vi "Initialise Sound From File.vi"(8 "error in (no error)":errorcluster, 10 "Name":string, 11 "File":path) -> (0 "error out":errorcluster, 3 "Name In Cache":string)   [LabVIEW 2015, in "Resource Manager.lvclass"]
uses:
  Resource Manager.lvclass
  Resource Manager.lvclass/Resource Manager.ctl
  Globals.vi
  LabSDL2/Source/Libraries/LibSDL2_Mixer Wrapper/LibSDL2_Mixer.lvlib
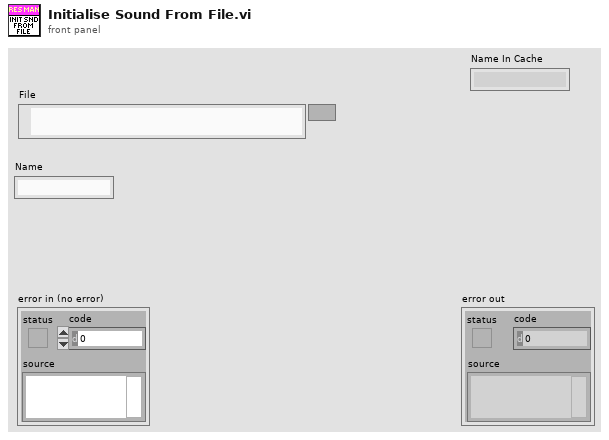
[diagram p1: front panel]
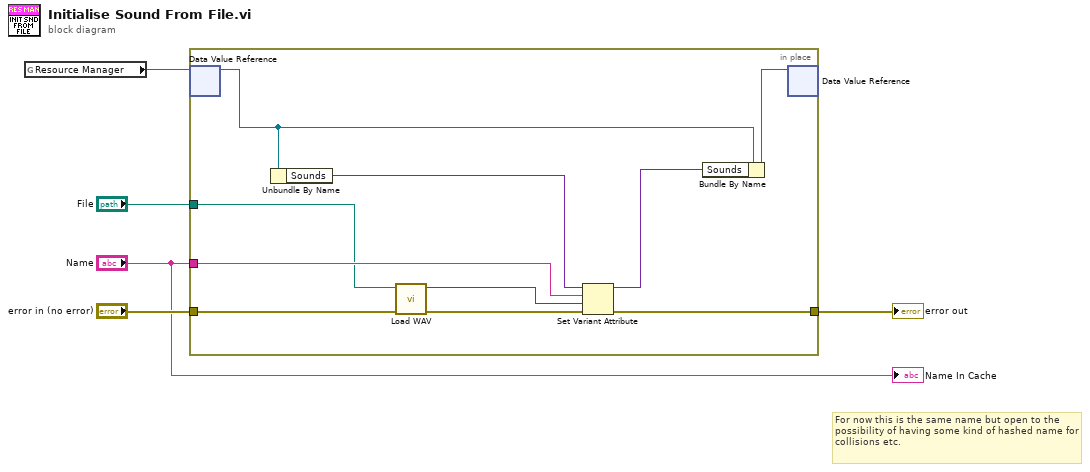
[diagram p0: block diagram]
diagram:
  # "For now this is the same name but open to the possibility of having some kind of hashed name for collisions etc."
  n1 = global read "Globals.vi" "Resource Manager"() -> (w1:refnum<data-value>)
  n2 = in-place {
    in-place-border: "File" -> [w7]
    in-place-border: "error in (no error)" -> [w9]
    in-place-border: [w14] -> w3
    in-place-border: "Name" -> [w12]
    n3 = in-place-dvr #1(w1) -> (w11:refnum<class "Resource Manager.lvclass">)  [unwired: 1 out]
    n4 = Unbundle By Name(w11) -> ("Sounds"=w15:variant)
    n5 = call "Load WAV.vi"("error in"=w9, "File"=w7) -> ("error out"=w8:errorcluster, "Chunk Pointer"=w6:u32)  [unwired: 8 in]
    n6 = Set Variant Attribute(Variant=w15, name=w12, value=w6, error in=w8) -> (Variant out=w13:variant, error out=w14:errorcluster)  [unwired: 1 out]
    n7 = Bundle By Name(cluster=w11, "Sounds"=w13) -> (w10:refnum<class "Resource Manager.lvclass">)
    n8 = in-place-dvr #1(w10) -> ()  [unwired: 2 out]
  }
  "error out" <- w3
  "Name In Cache" <- "Name"
